vi "DataProcess2.vi"(0 "DIO Group 1":T1={"Channel 1"=0, "Enable"=TRUE, "Main Switch"=0, "Channel 2"=0, "Channel 9"=0, "Channel 10"=0, "Channel 11"=0, "Channel 3"=0, "Channel 4"=0, "Channel 12"=0, "Channel 5"=0, "Channel 13"=0, "Channel 6"=0, "Channel 14"=0, "Channel 7"=0, "Channel 15"=0, "Channel 8"=0, "Channel 16"=0} caption="Data In") -> (1 "High":u16, 2 "Low":u16)   [LabVIEW 2012]
uses:
  ChannelStateControl.ctl
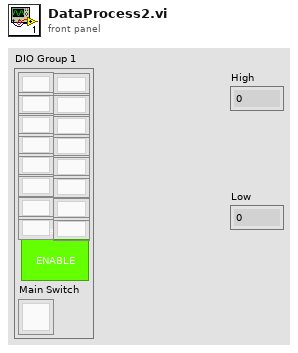
[diagram p1: front panel]
types:
  T1 = typedef "ChannelStateControl.ctl" = cluster{"Channel 1":u8, "Enable":bool, "Main Switch":u8, "Channel 2":u8, "Channel 9":u8, "Channel 10":u8, "Channel 11":u8, "Channel 3":u8, "Channel 4":u8, "Channel 12":u8, "Channel 5":u8, "Channel 13":u8, "Channel 6":u8, "Channel 14":u8, "Channel 7":u8, "Channel 15":u8, "Channel 8":u8, "Channel 16":u8}
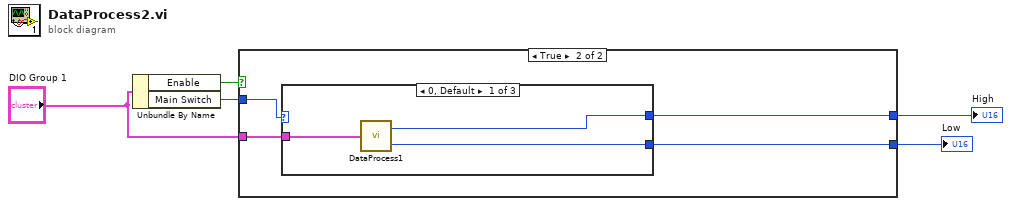
[diagram p0: block diagram]
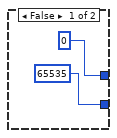
[diagram p2: hidden frame]
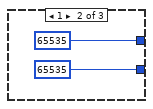
[diagram p3: hidden frame]
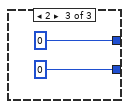
[diagram p4: hidden frame]
diagram:
  n1 = Unbundle By Name("DIO Group 1") -> ("Enable"=w5:bool, "Main Switch"=w4:u8)
  n2 = case shown="True" w5 {
    tunnel: [u16 0 w9] -> w2
    tunnel: [u16 65535 w8] -> w1
    tunnel: w4 -> [_ w11]
    tunnel: "DIO Group 1" -> [_ w10]
    frame False {
    }
    frame True {
      n3 = case shown="0, Default" w11 {
        tunnel: w10 -> [w12 _ _]
        tunnel: [w14 u16 65535 u16 0] -> w9
        tunnel: [w13 u16 65535 u16 0] -> w8
        frame 0, Default {
          n4 = call "DataProcess1.vi"("DIO Group 1"=w12) -> ("High Out"=w14:u16, "Low Out"=w13:u16)
        }
        frame 1 {
        }
        frame 2 {
        }
      }
    }
  }
  "High" <- w2
  "Low" <- w1
